vi "StimParam2String.vi"(1 "stimulus parameters":T1) -> (0 "serialized string":string)   [LabVIEW 2014]
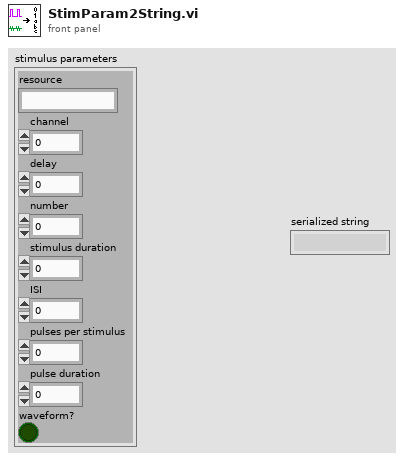
[diagram p1: front panel]
types:
  T1 = cluster{"resource":string, "channel":u16, "delay":dbl, "number":i32, "stimulus duration":dbl, "ISI":dbl, "pulses per stimulus":u16, "pulse duration":dbl, "waveform?":bool}
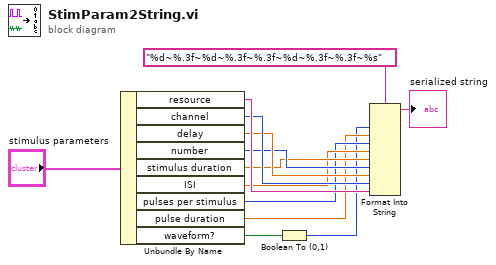
[diagram p0: block diagram]
diagram:
  n1 = Unbundle By Name("stimulus parameters") -> ("resource"=w11:string, "channel"=w10:u16, "delay"=w9:dbl, "number"=w8:i32, "stimulus duration"=w7:dbl, "ISI"=w6:dbl, "pulses per stimulus"=w5:u16, "pulse duration"=w4:dbl, "waveform?"=w3:bool)
  n2 = Boolean To (0,1)(Boolean=w3) -> (0, 1=w2:i16)
  n3 = Format Into String(format string="%d~%.3f~%d~%.3f~%.3f~%d~%.3f~%.3f~%s", w2, w4, w5, w6, w7, w8, w9, w10, w11) -> (resulting string=→"serialized string":string)  [unwired: 2 in, 1 out]
